vi "Part 2.vi"(11 "Input":string) -> (3 "Output":u64)   [LabVIEW 2021]
uses:
  <userlib>/_OpenG.lib/string/string.llb/Convert EOLs (String)__ogtk.vi
panel:
  in  "Input 2":string
  out "array 2":string[](array[string])
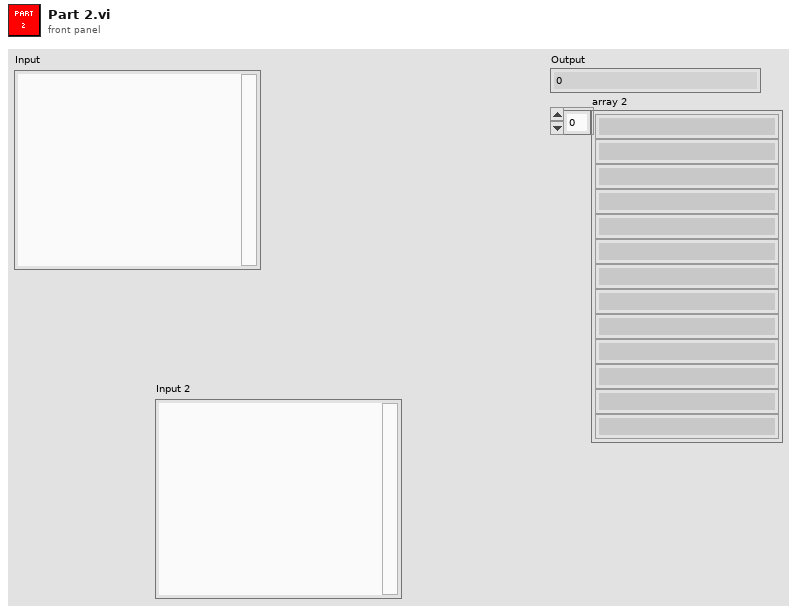
[diagram p1: front panel]
types:
  T1 = map{string, cluster{"Left":string, "Right":string}}
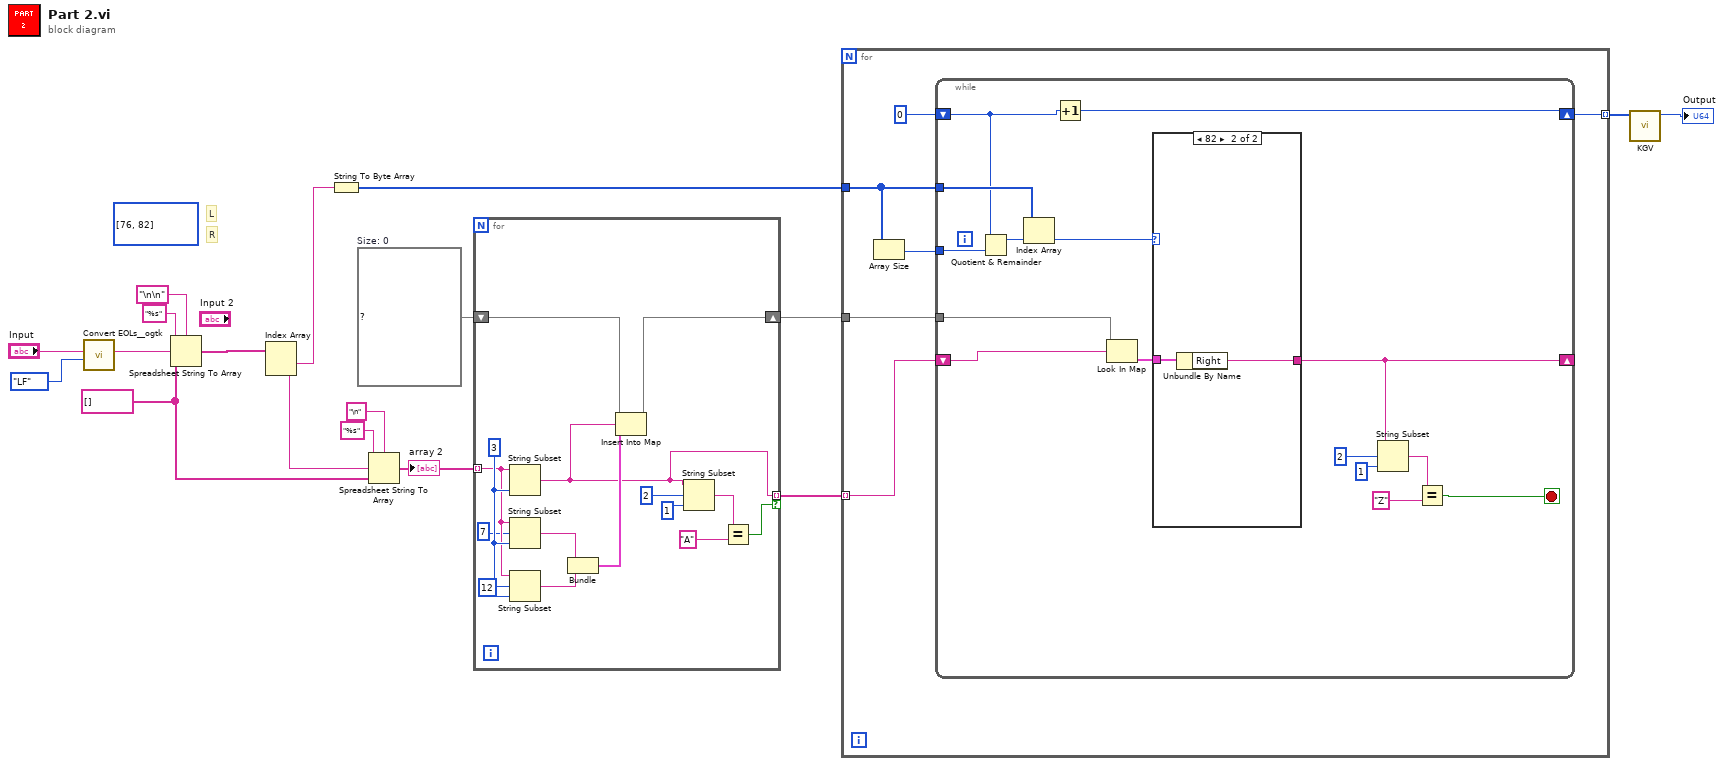
[diagram p0: block diagram]
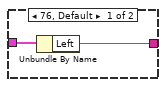
[diagram p2: hidden frame]
diagram:
  w6 = T1 {}  # Size: 0
  (unwired) u8[] [76, 82] ("unsigned byte array")
  w8 = string[] []
  # "R"
  # "L"
  n1 = call-poly <userlib>:"Convert EOLs__ogtk.vi"("Convert to:"=enum16{"CR", "LF", "CRLF"}."LF", "String in"="Input") -> ("String out"=w15:string)  [unwired: 9 in]
  n2 = Spreadsheet String To Array(delimiter (Tab)="\n\n", format string="%s", spreadsheet string=w15, array type (2D Dbl)=w8) -> (array=w13:string[])
  n3 = Index Array(array=w13) -> (element #1=w12:string, element #2=w9:string)  [unwired: 2 in]
  n4 = String To Byte Array(string=w12) -> (unsigned byte array=w3:u8[])
  n5 = Spreadsheet String To Array(delimiter (Tab)="\n", format string="%s", spreadsheet string=w9, array type (2D Dbl)=w8) -> (array=w7:string[])
  "array 2" <- w7
  n6 = for {
    tunnel: w7 -> [w32] mode=indexing
    shift-right: [w25] -> w5
    shift-left: w6 -> [w27]
    tunnel: [w20] -> w4 mode=indexing if=w21
    w33 = 3
    n7 = String Subset(string=w32, length (rest)=w33) -> (substring=w20:string)  [unwired: 1 in]
    n8 = String Subset(string=w32, offset (0)=7, length (rest)=w33) -> (substring=w28:string)
    n9 = String Subset(string=w32, offset (0)=12, length (rest)=w33) -> (substring=w29:string)
    n10 = Bundle(w28, w29) -> (w26:cluster{string, string})  [unwired: 1 in]
    n11 = Insert Into Map(map in=w27, key=w20, value=w26) -> (map out=w25:T1)  [unwired: 2 out]
    n12 = String Subset(string=w20, offset (0)=2, length (rest)=1) -> (substring=w19:string)
    n13 = Equal?(x=w19, y="A") -> (x = y?=w21:bool)
  }
  n14 = for {
    tunnel: w5 -> [w39]
    tunnel: w4 -> [w37] mode=indexing
    tunnel: w3 -> [w36]
    tunnel: [w34] -> w2 mode=indexing
    n15 = Array Size(array=w36) -> (size(s)=w38:i32)
    n16 = while {
      tunnel: w38 -> [w54]
      tunnel: w36 -> [w52]
      shift-right: [w48] -> _
      shift-left: w37 -> [w49]
      tunnel: w39 -> [w50]
      shift-right: [w46] -> w34
      shift-left: u64 0 -> [w47]
      stop <- w40 stop-if-true
      n17 = Quotient & Remainder(x=w47, y=w54) -> (x-y*floor(x/y)=w53:u64)  [unwired: 1 out]
      n18 = Index Array(array=w52, index=w53) -> (element=w51:u8)
      n19 = Increment(x=w47) -> (x+1=w46:u64)
      n20 = Look In Map(map=w50, key=w49) -> (value=w45:cluster{"Left":string, "Right":string})  [unwired: 1 in, 1 out]
      n21 = case shown="82" w51 {
        tunnel: w45 -> [w56 w58]
        tunnel: [w55 w57] -> w48
        frame 76, Default {
          n22 = Unbundle By Name(w56) -> ("Left"=w55:string)
        }
        frame 82 {
          n23 = Unbundle By Name(w58) -> ("Right"=w57:string)
        }
      }
      n24 = String Subset(string=w48, offset (0)=2, length (rest)=1) -> (substring=w41:string)
      n25 = Equal?(x=w41, y="Z") -> (x = y?=w40:bool)
    }
  }
  n26 = call "KGV.vi"("Array"=w2) -> ("KGV"=→"Output":u64)  [unwired: 10 in]
